vi "Read Y.vi"(8 "error in (no error)":errorcluster, 11 "VISA Refnum in":refnum<visa-resource-name>) -> (0 "error out":errorcluster, 1 "Wavelike Data":dbl[](array[numeric]), 2 "Return All Data":string, 3 "VISA Refnum out":refnum<visa-resource-name>, 7 "Return Data Bytes":u16)   [LabVIEW 2018]
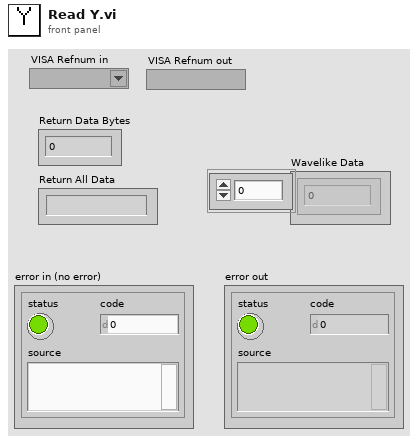
[diagram p1: front panel]
types:
  T1 = enum16{"Y AXIS Data Output", "X AXIS Data Output"}
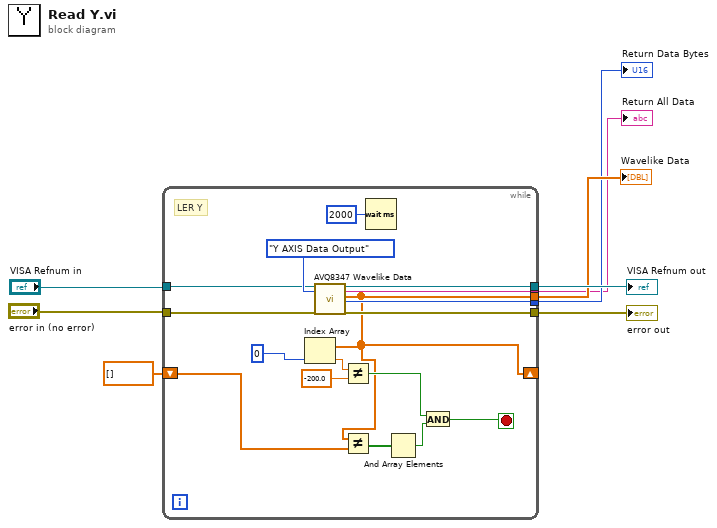
[diagram p0: block diagram]
diagram:
  n1 = while {
    tunnel: [w24] -> w2
    tunnel: [w23] -> w3
    tunnel: [w13] -> w4
    tunnel: "VISA Refnum in" -> [w19]
    tunnel: [w22] -> w7
    tunnel: "error in (no error)" -> [w20]
    tunnel: [w21] -> w8
    shift-right: [w13] -> _
    shift-left: dbl[] [] ("Wavelike Data") -> [w12]
    stop <- w9 stop-if-true
    # "LER Y"
    n2 = call "AVQ8347 Wavelike Data.vi"("VISA Session"=w19, "Axis Select"=T1."Y AXIS Data Output", "Error In"=w20) -> ("Copy VISA Session"=w22:refnum<visa-resource-name>, "Return All Data"=w24:string, "Wavelike Data"=w13:dbl[], "Return Data Bytes"=w23:u16, "Error Out"=w21:errorcluster)  [unwired: 12 in]
    n3 = Index Array(array=w13, index=0) -> (element=w15:dbl)
    n4 = Not Equal?(x=w15, y=-200.0) -> (x != y?=w14:bool)
    n5 = Not Equal?(x=w13, y=w12) -> (x != y?=w11:bool[])
    n6 = Wait (ms)(milliseconds to wait=u32 2000) -> ()  [unwired: 1 out]
    n7 = And Array Elements(Boolean array=w11) -> (logical AND=w10:bool)
    n8 = And(x=w14, y=w10) -> (x .and. y?=w9:bool)
  }
  "error out" <- w8
  "VISA Refnum out" <- w7
  "Wavelike Data" <- w4
  "Return Data Bytes" <- w3
  "Return All Data" <- w2
